vi "SetForceBurst.vi"(8 "error in (no error)":errorcluster, 11 "config":T1) -> (0 "error out":errorcluster, 3 "config out":T1)   [LabVIEW 2017, in "BurstMode.lvlib"]
uses:
  <vilib>/addons/InsightCM/Devices/Shared/Cms/CmsBurstMode/BurstMode.lvlib
  <vilib>/addons/InsightCM/Devices/Shared/Cms/CmsBurstMode/controls/config.ctl
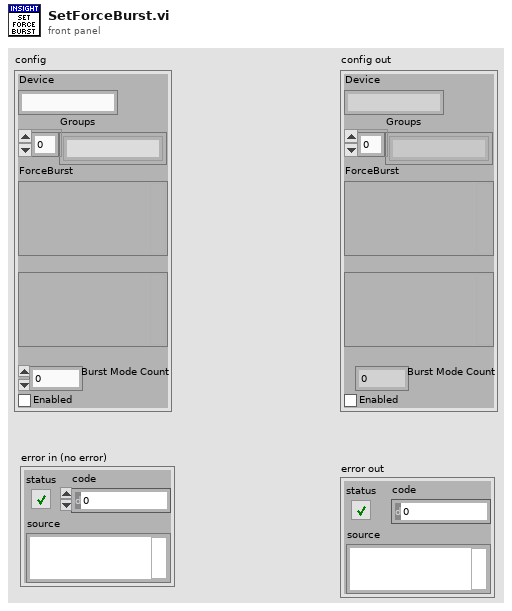
[diagram p1: front panel]
types:
  T1 = typedef "BurstMode.lvlib/config.ctl" = cluster{"Device":string, "Groups":string[], "ForceBurst":variant, "TriggerBurst":variant, "Burst Mode Count":i32, "Enabled":bool}
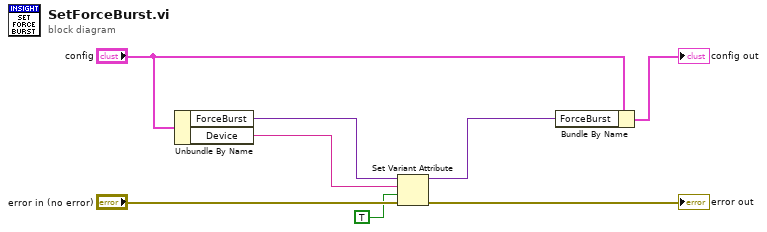
[diagram p0: block diagram]
diagram:
  n1 = Unbundle By Name("config") -> ("ForceBurst"=w2:variant, "Device"=w3:string)
  n2 = Set Variant Attribute(Variant=w2, name=w3, value=TRUE ("ForceTrigger"), error in="error in (no error)") -> (Variant out=w6:variant, error out=→"error out":errorcluster)  [unwired: 1 out]
  n3 = Bundle By Name(cluster="config", "ForceBurst"=w6) -> (→"config out":T1)
